vi "2024_day01.vi"() -> ()   [LabVIEW 2023]
uses:
  <userlib>/_OpenG.lib/array/array.llb/Search 1D Array (I32)__ogtk.vi
  <userlib>/_OpenG.lib/string/string.llb/openg_string.lvlib
  <userlib>/_OpenG.lib/array/array.llb/openg_array.lvlib
panel:
  out "Result - Task 2":i32
  out "Result - Task 1":i32
  in  "Switch":bool caption="Ex. Data  vs.  User Data"
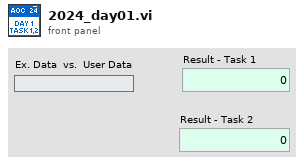
[diagram p1: front panel]
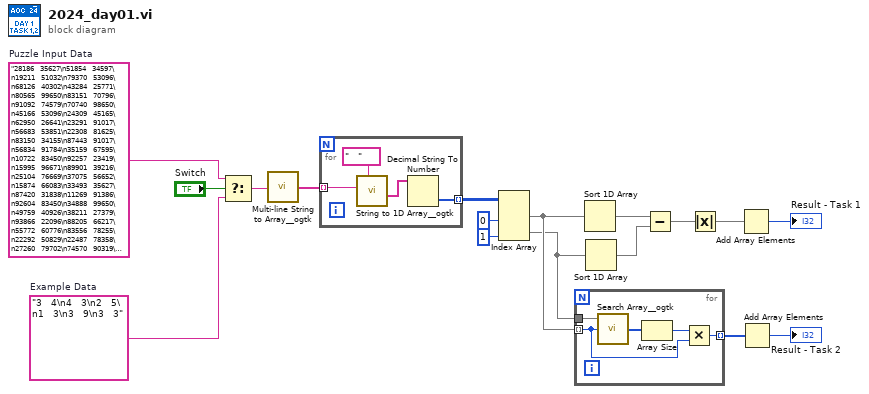
[diagram p0: block diagram]
diagram:
  w15 = "28186   35627\n51854   34597\n19211   51032\n79370   53096\n68126   40302\n43284   25771\n80565   99650\n83151   70796\n91092   74579\n70740   98650\n45166   53096\n24309   45165\n62950   26641\n23291   91017\n56683   53851\n22308   81625\n83150   34155\n87443   91017\n56834   91784\n35159   67595\n10722   83450\n92257   23419\n15995   96671\n89901   39216\n25104   76669\n37075   56652\n15874   66083\n33493   35627\n87420   31838\n11269   91386\n92604   83450\n34888   99650\n49759   40926\n38211   27379\n93866   22096\n88205   66217\n55772   60776\n83556   78255\n22292   50829\n22487   78358\n27260   79702\n74570   90319\n27532   14353\n40720   67595\n99885   65688\n25733   53752\n12466   14411\n88402   40165\n63328   13804\n45165   62461\n24913   94225\n32251   76669\n91004   40165\n48939   45165\n98082   34561\n74569   42932\n99641   54600\n42748   22021\n23376   54490\n38706   69865\n64985   87783\n14431   78715\n37671   94814\n27425   60776\n21801   76669\n96975   33493\n56680   31838\n41265   71129\n99081   32487\n53077   82615\n54490   55624\n22649   60776\n82601   25943\n93133   96412\n77182   78358\n67827   76838\n45976   89107\n20352   89034\n28891   23800\n87739   76669\n47802   99650\n18060   28437\n65882   93980\n53343   13764\n84301   93604\n62547   93479\n79067   45165\n70139   54490\n28158   76669\n71631   39775\n36521   57540\n78928   37888\n75943   39076\n28462   60107\n95828   94225\n49768   73181\n40545   97945\n18963   74260\n17934   63046\n73054   13454\n43170   60924\n90257   28180\n99765   33493\n41380   50296\n24225   62945\n66579   73961\n73361   54622\n26339   91017\n84080   62041\n89322   54600\n84610   18344\n58420   87051\n12253   83450\n25631   91017\n71764   63533\n52908   40165\n56578   46636\n99876   61946\n43934   64469\n78242   11111\n97629   28916\n21477   91017\n97639   64456\n90978   53077\n94412   73836\n49249   96113\n92750   14411\n12961   13764\n84319   22230\n83435   78146\n48951   86109\n40258   13764\n54600   65577\n51432   53096\n11527   20394\n68196   94225\n14939   91017\n13158   39216\n62120   93587\n20939   71764\n58436   28038\n37198   31838\n59152   17554\n52958   44145\n64236   18285\n63763   56578\n40304   99650\n86564   78910\n45684   52760\n43139   61946\n99974   76669\n44698   86004\n19940   22021\n29106   78358\n60431   91386\n50880   76451\n96595   42193\n40966   73961\n64515   61946\n31081   39834\n87614   70892\n82663   54622\n73537   62994\n14125   56652\n51361   35627\n26084   35817\n82915   20069\n72409   22021\n22834   20071\n93476   83787\n63719   53096\n41505   48056\n56055   20404\n37255   99650\n33468   60776\n70472   22598\n66290   53077\n91071   67595\n30888   33173\n60826   29871\n12334   78358\n62744   69424\n85449   79500\n22333   16295\n67621   18455\n12605   90059\n32490   25835\n96639   75870\n82412   39747\n76964   60153\n60776   60776\n68837   39216\n35635   67595\n85239   14964\n15278   83450\n63581   35178\n77006   18285\n88570   80424\n61499   81689\n57466   47392\n78524   84304\n11821   53989\n62425   28916\n36264   50872\n38567   13061\n16357   45165\n17202   94451\n64290   31838\n76075   55071\n87325   40165\n93961   99650\n49866   65601\n91725   14411\n44721   18285\n44065   33493\n22521   56578\n28070   54600\n45621   54600\n54677   26913\n79647   24298\n89613   31415\n86493   13764\n16243   64218\n12832   21187\n43847   35189\n75859   54600\n69276   75826\n43251   14411\n96012   41446\n35482   35817\n45380   82383\n66801   31838\n79199   92341\n33087   70511\n40619   28916\n67655   80670\n22431   60776\n62731   54622\n29873   25771\n99354   63481\n36415   61946\n29742   94919\n64872   53077\n93028   55635\n32784   18285\n87488   68734\n56652   18285\n49968   80712\n82653   53096\n30377   24784\n40120   45165\n88404   70120\n69179   45165\n99645   67595\n44883   45165\n76320   43595\n29057   90019\n28502   61946\n73459   84304\n96354   54622\n77589   14301\n51381   54490\n40490   95808\n36023   27135\n13434   63807\n27250   35627\n13764   32845\n28229   34954\n56430   76669\n98593   63811\n11192   60776\n81601   72265\n86908   77116\n25484   82383\n31115   42206\n75124   70148\n96785   53096\n59814   85995\n17024   57255\n81701   41971\n43938   33493\n91646   33599\n96616   81828\n73270   87775\n75876   35817\n53007   83450\n39527   33975\n35936   17039\n95194   23302\n96876   80147\n68136   91386\n31253   19760\n98767   61208\n98353   86604\n13239   36264\n43374   13764\n36658   22965\n58030   84304\n42686   78358\n99419   49423\n43976   20759\n33361   47852\n23794   61946\n26896   83450\n12213   37740\n53827   49270\n71874   61946\n19394   77889\n63728   81025\n63780   72467\n34161   21317\n81832   56652\n20986   99650\n36631   48302\n60232   63009\n37744   84304\n46964   39391\n19771   14411\n75783   69365\n71727   71252\n60541   69095\n68594   30949\n51619   88697\n26797   50216\n86654   61946\n98872   53347\n20079   18807\n60408   41952\n37203   47862\n92078   43717\n94853   53096\n91937   65490\n39800   79198\n14179   50429\n21846   72768\n19081   14411\n60170   39838\n14482   36264\n61946   64811\n88464   10899\n93401   44867\n42260   53495\n92730   76838\n17708   31838\n68523   99650\n44540   95629\n12785   54490\n34598   13764\n20161   28916\n15318   67595\n67423   47864\n13951   95495\n63011   67595\n73505   61946\n22300   73685\n35181   78358\n70531   60776\n95954   57049\n65463   67851\n67270   53593\n62726   13782\n66690   72865\n99591   33493\n89300   13764\n82383   51267\n55326   56578\n66315   54622\n51554   91145\n21778   67595\n38569   71437\n25915   80353\n92411   88336\n76148   83204\n68688   61443\n78063   34003\n27804   14411\n79316   59050\n14222   22021\n83018   18197\n36304   33795\n46381   78358\n23167   99650\n73696   11314\n83569   71391\n93902   76551\n33606   35906\n30257   54600\n24956   80860\n64619   14411\n17640   56652\n22908   83696\n18954   74347\n89497   83450\n70303   76669\n37979   69814\n22661   53077\n96573   83961\n13055   85059\n73265   67595\n31927   45165\n61607   54490\n62232   53096\n68738   79113\n50586   95006\n55731   39122\n33386   31838\n20118   97657\n98794   76669\n62869   57813\n45508   91386\n29960   56652\n20228   95663\n75424   74090\n75421   30158\n82307   11086\n26488   64910\n48430   41174\n81439   63107\n68896   56652\n67511   33375\n40446   66170\n13668   68369\n83234   16181\n16929   84304\n42735   85915\n93954   22403\n98252   33493\n39418   54622\n14183   89745\n67167   68002\n88731   22021\n42317   54490\n29404   83450\n80844   31838\n43255   34866\n61762   32538\n32255   78358\n93152   25771\n42141   56578\n83740   22021\n40030   47353\n34668   14411\n46752   21905\n26196   48915\n45243   67595\n26757   56652\n13969   82383\n13148   84304\n39362   29711\n92819   31171\n12210   14411\n58671   91017\n87279   62713\n97755   92124\n77086   62944\n87094   40099\n83398   35817\n36525   64734\n27346   36264\n50274   17587\n74438   92593\n86182   13764\n63946   56578\n99269   25771\n46815   67595\n44645   93146\n82027   25771\n46981   39216\n52039   31814\n25930   54600\n48743   31838\n80123   72281\n21790   84579\n91556   78358\n63961   14411\n11280   97891\n67372   60776\n35817   34731\n80767   53877\n32458   90108\n53471   13557\n76699   92723\n33967   31838\n83166   23325\n48974   44826\n28408   16412\n18980   61946\n76595   21581\n54278   82835\n57836   67595\n16791   84304\n52746   99650\n23543   83450\n28819   95078\n21590   84304\n90588   91017\n62879   43669\n35788   81389\n67595   91386\n43342   73961\n34072   73961\n41533   54487\n77769   71151\n95215   74006\n37630   44436\n85291   18292\n82845   99650\n56633   60776\n95645   54490\n59689   14411\n77873   23174\n47892   94225\n71442   77808\n52932   56578\n68699   56652\n70296   54600\n34780   50848\n14008   63408\n65865   73961\n64689   84695\n70986   45490\n20034   54600\n21194   73961\n42510   37716\n80906   32357\n38289   19304\n44371   53386\n45873   95639\n72359   53096\n26200   40165\n81093   32591\n75520   99689\n70526   92020\n38000   90543\n42109   40526\n65858   64811\n77533   83450\n84191   63489\n59480   46311\n20750   32879\n81791   76258\n49948   56739\n44960   22021\n49084   12978\n46948   25438\n22467   39216\n32066   41311\n47715   13764\n40689   56652\n81797   82792\n48102   91114\n13286   64910\n24324   81079\n14772   91386\n10721   20481\n26990   54622\n67169   22021\n42848   25771\n24672   13764\n86122   25771\n56904   13764\n81436   53096\n94624   33493\n91853   56652\n23675   14088\n26625   68877\n22777   53096\n44833   33493\n47549   96449\n79529   27951\n78188   99650\n16287   51001\n64231   25771\n84131   55907\n15378   41016\n69506   78358\n80392   64811\n68681   57430\n95565   40165\n27128   40839\n11911   38020\n32463   95974\n64051   39216\n59409   25771\n85311   99650\n15025   76669\n31085   83450\n57046   43589\n31356   25944\n53445   32566\n65374   24456\n94347   17250\n51998   76838\n38930   76838\n13223   22328\n23412   33493\n33498   39216\n66922   97888\n19340   13764\n30800   33625\n63834   53077\n26329   76669\n36202   52321\n99460   87180\n10752   22155\n83677   54586\n83136   94225\n43505   94775\n49792   51024\n18430   87697\n48959   62169\n27559   86092\n42055   71266\n47346   27875\n95130   15327\n67175   50520\n80717   48669\n98758   93010\n69621   73606\n25596   22021\n37015   83450\n14944   93706\n70867   84304\n14464   80652\n11365   25771\n78435   46797\n45002   58808\n57900   83487\n99650   55843\n80681   38011\n64811   86071\n97586   33898\n42094   41087\n76669   54622\n74600   28060\n18109   25771\n95834   40165\n76583   32274\n23271   54600\n73123   81744\n81442   70437\n97274   25771\n99106   91717\n19847   39216\n41705   54622\n97824   64338\n34982   39216\n47246   58999\n94716   78358\n52266   60776\n39216   95154\n49351   94864\n64910   39559\n43455   84248\n71500   27152\n30651   49103\n63267   44712\n17567   18998\n63046   48579\n51483   63529\n35182   14411\n73961   60776\n39993   30182\n26258   96243\n52698   77762\n21525   22021\n47513   20331\n13140   22021\n43778   40165\n22788   94225\n84367   31838\n54265   64910\n55305   42377\n78923   54586\n40429   39216\n12422   63046\n24878   94225\n64356   57593\n34812   40889\n54661   60776\n31004   55132\n38061   63046\n85827   35627\n72862   33704\n51636   98691\n15448   54159\n90048   67595\n53851   18285\n48530   74924\n20386   81637\n87273   53096\n83022   56018\n98251   65250\n89295   60776\n98142   15765\n31571   42354\n92874   70979\n44965   58401\n51688   78358\n93890   12104\n65530   53096\n55006   91017\n49672   55977\n31815   37826\n13567   58321\n60844   53077\n63845   26325\n98712   79314\n99601   63236\n14173   60776\n11249   86708\n37023   48603\n25248   14411\n25444   63817\n92822   10083\n43060   41903\n98283   89972\n10004   77190\n69379   56652\n30459   45165\n81481   18285\n47130   24016\n57377   56872\n24043   63046\n78319   33493\n96058   33493\n42928   32466\n76838   35627\n43659   76669\n36827   39216\n41007   60776\n79655   14411\n26608   44836\n85420   68185\n81174   96069\n79223   59880\n54106   52192\n71917   83450\n19775   73961\n45391   66102\n26838   33493\n53437   76669\n71922   91017\n67552   40770\n23842   12889\n75398   90858\n20264   96094\n38278   39216\n62780   68287\n92766   45165\n25677   23355\n55791   83450\n63556   93703\n97511   61946\n74712   18285\n34605   15067\n57436   56652\n91202   91017\n11656   54622\n31838   22156\n94443   25771\n84090   60590\n63298   91386\n60339   56419\n25780   53096\n55284   76669\n83080   71920\n53843   36881\n83616   42743\n89091   68085\n71899   31838\n57786   67595\n34559   96506\n77211   94225\n67812   61946\n26511   63739\n51963   97847\n81350   23053\n37978   57093\n93413   89804\n38133   60776\n73234   84629\n60624   31957\n13937   34269\n35804   44626\n36210   53096\n34190   33493\n30736   83057\n80091   23762\n60917   82383\n30227   53096\n94439   56652\n78308   67595\n51009   67595\n64010   53077\n20563   61946\n43967   17312\n86436   75180\n80389   42825\n94453   83450\n41805   91918\n21462   99650\n71157   10537\n35046   73961\n96103   74733\n83069   35732\n18285   82383\n26446   76669\n70874   18579\n10539   11666\n57999   83450\n25966   91017\n37570   93089\n46126   18897\n65025   78341\n48404   61946\n26116   91017\n84857   33493\n84369   96112\n79609   76561\n24415   76669\n55288   37007\n85869   10010\n15152   76669\n10609   52954\n56293   59754\n35563   99650\n15144   32125\n27560   33493\n10484   99261\n73264   74795\n44774   17094\n41294   53851\n14411   83990\n17065   25771\n25771   60026\n58907   16393\n93527   90760\n25715   68223\n61620   23456\n36485   15169\n70191   39216\n40165   94225\n54006   99650\n75597   53096\n49678   25771\n51574   96842\n57852   18285\n60104   61946\n78607   35627\n54889   14411\n47241   10303\n71456   94225\n81425   49149\n59061   28602\n24633   31838\n14420   93613\n54622   53077\n17040   78745\n70622   88133\n56992   72730\n97895   33493\n94648   44310\n59138   13764\n97350   69918\n32734   83579\n55320   66823\n96915   55216\n95293   38588\n13774   12822\n70053   58437\n22021   18724\n41216   43315\n28987   31838\n70488   89770\n48277   53914\n79376   76669\n94225   53077\n60803   12578\n21144   16837\n23645   33714\n28916   83751\n50535   31838\n62178   64811\n63126   71848\n33569   46461\n99826   53077\n74714   33856\n67967   26838\n83610   54622\n15872   36009\n34302   31838\n24069   56292\n90147   38554\n95987   79195\n62656   40165\n83153   26094\n68726   85767\n63172   74949\n35390   94225\n29379   63046\n13571   56578\n16169   64811\n68905   35817\n71763   53096\n48781   28841\n95966   15028\n87862   67072\n87176   60776\n11203   13761\n50294   11171\n21503   25547\n96570   78358\n25213   84422\n61744   85120\n62795   72393\n84907   33493\n82935   84304\n24224   36264\n91386   99650\n76217   98074\n73872   60776\n41777   19177\n95695   39216\n88779   15111\n93458   67595\n74732   67770\n23754   39216\n90662   35817\n24013   99650\n66779   83450\n54586   27524\n88285   69874\n47809   22021\n25662   71764\n31583   56652\n58156   60776\n22656   56578\n22315   76174\n70195   54622\n27027   33351\n32409   75991\n91017   72493\n53096   13301\n92656   41863\n84304   85568\n45081   73961\n21844   78358\n83024   61946\n93888   45113\n69174   53096\n98465   56543\n46208   56652\n63289   99650\n96607   76329\n62648   55561\n38090   62481\n87491   90246\n45019   81753\n88050   73961\n18142   26270\n36682   22021\n15933   94225\n17393   38533\n33633   67595\n55662   73961\n63567   74739\n69557   83450\n36169   25771\n40716   35837\n11665   14704\n94437   36515\n43859   18285\n98937   54490\n73932   94209\n99289   50655\n12403   22021\n80283   64811\n68700   43336\n36887   69617\n53551   83450\n76290   18285\n49743   25771\n35627   76669\n59070   13231\n40419   24169\n48544   82383\n68680   84304\n31610   58761\n31170   67595\n27004   41596\n62727   98757\n24189   76875\n42807   97581\n85552   71764\n52402   40046\n78358   41164\n83450   76669\n62947   25771\n55820   53096\n"  # Puzzle Input Data
  w16 = "3   4\n4   3\n2   5\n1   3\n3   9\n3   3"  # Example Data
  n1 = Select(t=w15, s="Switch", f=w16) -> (s? t:f=w14:string)
  n2 = call <userlib>:"Multi-line String to Array__ogtk.vi"("string"=w14) -> ("lines"=w13:string[])
  n3 = for {
    tunnel: w13 -> [w21] mode=indexing
    tunnel: [w18] -> w10 mode=indexing
    n4 = call <userlib>:"String to 1D Array__ogtk.vi"("delimiter (Tab)"="   ", "string"=w21) -> ("Array of Strings"=w19:string[])  [unwired: 9 in]
    n5 = Decimal String To Number(string=w19) -> (number=w18:i32[])  [unwired: 2 in, 1 out]
  }
  n6 = Index Array(array=w10, index (col) #1=0 ("disabled index (col)"), index (col) #2=1 ("index (col)")) -> (element #1=w4:i32[], element #2=w3:i32[])  [unwired: 2 in]
  n7 = for {
    tunnel: w4 -> [w22] mode=indexing
    tunnel: w3 -> [w26]
    tunnel: [w23] -> w2 mode=indexing
    n8 = call-poly <userlib>:"Search Array__ogtk.vi"("Array"=w26, "Element Data"=w22) -> ("Indices of Elements"=w25:i32[])  [unwired: 7 in]
    n9 = Array Size(array=w25) -> (size(s)=w24:i32)
    n10 = Multiply(x=w24, y=w22) -> (x*y=w23:i32)
  }
  n11 = Sort 1D Array(array=w4) -> (sorted array=w7:i32[])
  n12 = Sort 1D Array(array=w3) -> (sorted array=w6:i32[])
  n13 = Subtract(x=w7, y=w6) -> (x-y=w9:i32[])
  n14 = Absolute Value(x=w9) -> (abs(x)=w5:i32[])
  n15 = Add Array Elements(numeric array=w5) -> (sum=→"Result - Task 1":i32)
  n16 = Add Array Elements(numeric array=w2) -> (sum=→"Result - Task 2":i32)
